vi "set.vi"(7 "LabVIEW Web Service Request":refnum<class "Web Request.lvclass">) -> ()   [LabVIEW 2019]
uses:
  <vilib>/wsapi/Web Request.lvclass
panel:
  # "Use the Web Service Request input terminal to call the VIs on the Web Services palette. Do not remove it from the connector pane unless you don't need access to the palette."
  # "Each additional control wired to the connector pane will be available as an input in the URL. To include an indicator in terminal-mode output (the default setting), it must also be wired to the connector pane."
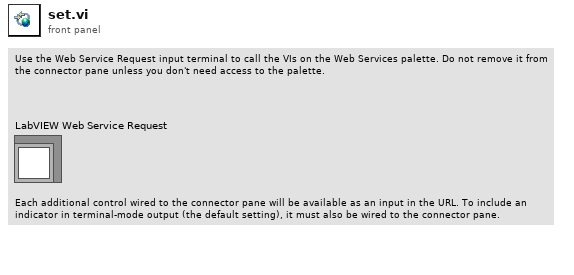
[diagram p1: front panel]
types:
  T1 = cluster{"[0]":string, "[1]":string, "[2]":string, "[3]":string}
  T2 = cluster{"[0]":errorcluster, "[1]":errorcluster, "[2]":errorcluster, "[3]":errorcluster}
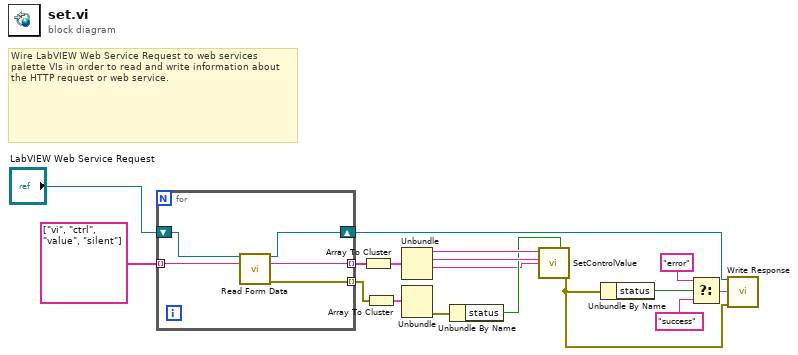
[diagram p0: block diagram]
diagram:
  # "Wire LabVIEW Web Service Request to web services palette VIs in order to read and write information about the HTTP request or web service."
  n1 = for {
    tunnel: string[] ["vi", "ctrl", "value", "silent"] -> [w21] mode=indexing
    tunnel: [w20] -> w12 mode=indexing
    shift-right: [w19] -> w2
    shift-left: "LabVIEW Web Service Request" -> [w18]
    tunnel: [w22] -> w9 mode=indexing
    n2 = call <vilib>:"Read Form Data.vi"("LabVIEW Web Service Request"=w18, "key"=w21) -> ("LabVIEW Web Service Request out"=w19:refnum<class "Web Request.lvclass">, "value"=w20:string, "error out"=w22:errorcluster)  [unwired: 10 in, 1 out]
  }
  n3 = Array To Cluster(array=w12) -> (cluster=w11:T1)
  n4 = Array To Cluster(array=w9) -> (cluster=w8:T2)
  n5 = Unbundle(w11) -> ("[0]"=w6:string, "[1]"=w5:string, "[2]"=w1:string)  [unwired: 1 out]
  n6 = Unbundle(w8) -> ("[3]"=w7:errorcluster)  [unwired: 3 out]
  n7 = Unbundle By Name(w7) -> ("status"=w4:bool)
  n8 = call "SetControlValue.vi"("vi"=w6, "Signaling"=w4, "ctrl"=w5, "Value (JSON)"=w1) -> ("error out"=w3:errorcluster)  [unwired: 11 in]
  n9 = Unbundle By Name(w3) -> ("status"=w16:bool)
  n10 = Select(t="error", s=w16, f="success") -> (s? t:f=w17:string)
  n11 = call <vilib>:"Write Response.vi"("LabVIEW Web Service Request"=w2, "response string"=w17, "error in (no error)"=w3) -> ()  [unwired: 11 in, 2 out]
